vi "Steruerungs Type erkennen.vi"(8 "error in (no error)":errorcluster caption="Fehler (Eingang, kein Fehler)", 10 "Steuerungs Type":i32[](array[numeric]), 11 "Steuerung PNS Eingang":refnum<class "Steuerung PNS.lvclass">) -> (0 "error out":errorcluster caption="Fehler (Ausgang)", 3 "Steuerung PNS Ausgang":refnum<class "Steuerung PNS.lvclass">)   [LabVIEW 2020, in "Steuerung PNS.lvclass"]
doc: "Hier wird tatsächlich die OjektKlasse je nach SteuerungsType gewechselt und schreibt diese ins Objekt (falls diese noch nicht gesetzt wrude oder nicht mehr den selben Wert hat - Tausch des PNS mit AutoDetection).\nRIW"
uses:
  Steuerung PNS.lvclass
  Steuerung PNS.lvclass/Steuerung PNS.ctl
  SteuerungsType (Enum).ctl
  Schneider Steuerung PNS/Schneider Steuerung PNS.lvclass
  D:/LabView_2020/LP und Compact Standardprogramm_20-10-14/ObjektKlassen/Steuerung PNS/Steuerung PNS.lvclass
  mini8 Steuerung PNS/mini8 Steuerung PNS.lvclass
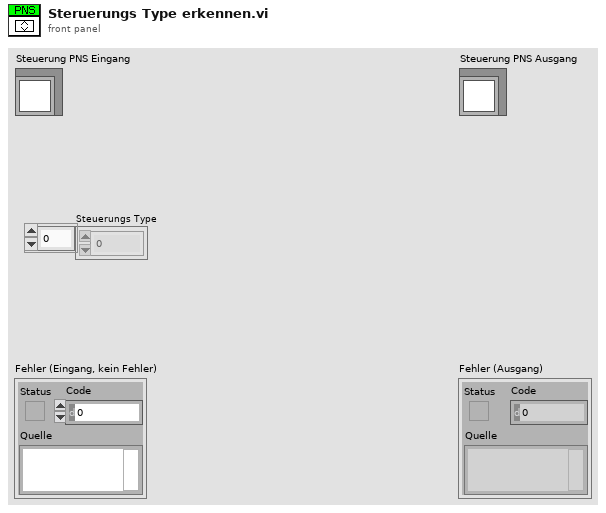
[diagram p1: front panel]
types:
  T1 = typedef "Steuerung PNS.lvclass/SteuerungsType (Enum).ctl" = enum16{"undefiniert", "Mini 8", "Schneider"}
  T2 = typedef "Steuerung PNS.lvclass/Anlegengrenzwerte PNS.ctl" = cluster{"Filter:":T3, "Ventilplatte:":T3, "Heizleitung 1:":T3, "Heizleitung 2:":T3, "Heizleitung 3:":T3, "Heizleitung 4:":T3, "Heizleitung 5:":T3, "Heizleitung 6:":T3}
  T3 = typedef "Steuerung PNS.lvclass/Anlagengrenzwerte Parameteranzeige.ctl" = cluster{"Sollwert":T4, "Warn-Min":T4, "Warn-Max":T4, "Abschalt-Min":T4, "Abschalt-Max":T4, "Regler":u16, "AnlagenParameter":string}
  T4 = typedef "Zahlen-Eingabefeld.ctl" = sgl
  T5 = typedef "Steuerung PNS.lvclass/Adresse.ctl" = cluster{i32[][], i32}
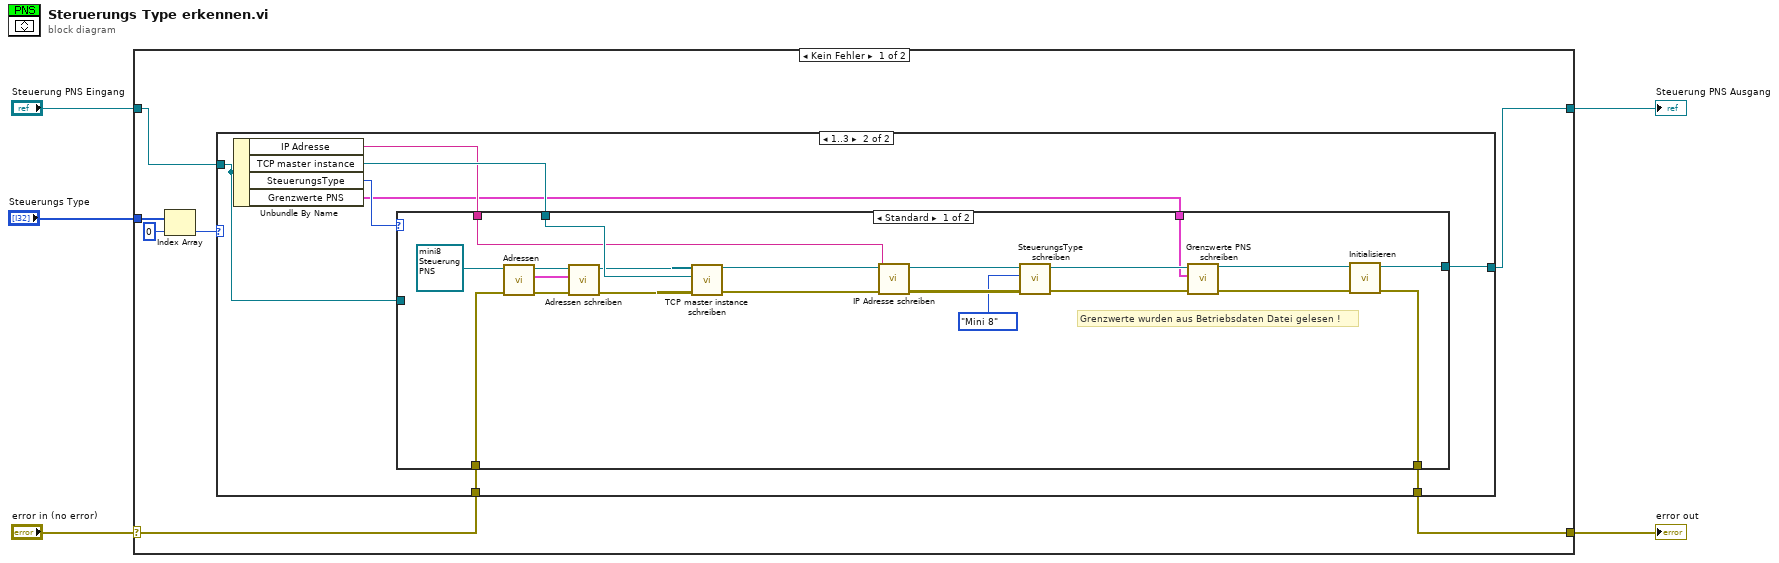
[diagram p0: block diagram]
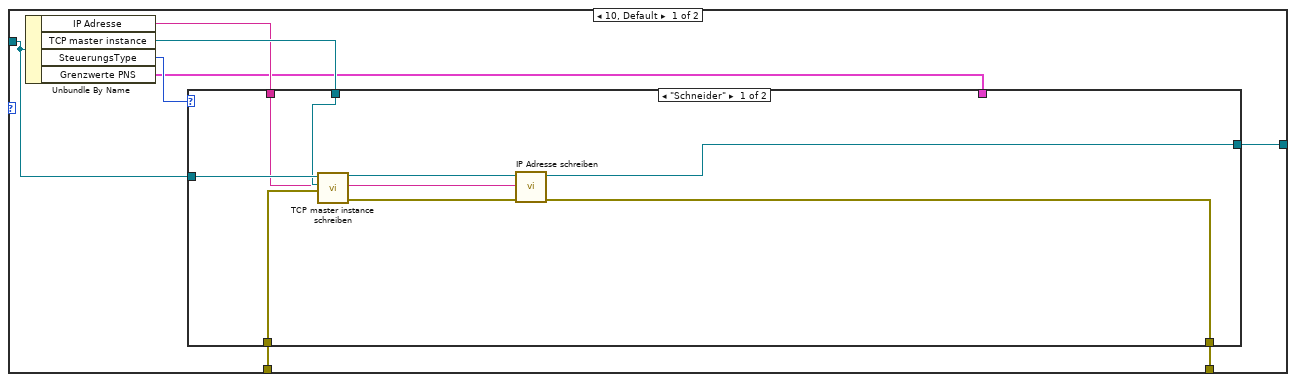
[diagram p2: hidden frame]
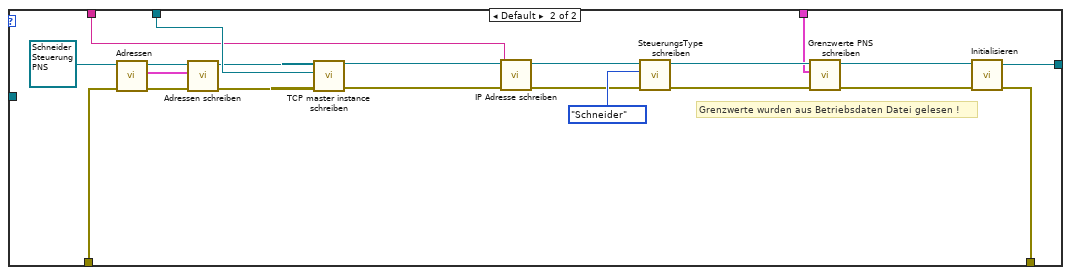
[diagram p3: hidden frame]
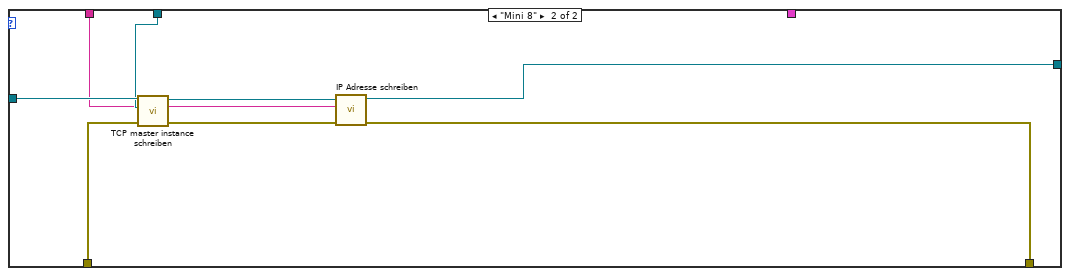
[diagram p4: hidden frame]
diagram:
  n1 = case shown="Kein Fehler" "error in (no error)" {
    selector: "error in (no error)" -> [w8 w86]
    tunnel: [w7 w86] -> w4
    tunnel: [w6 w85] -> w2
    tunnel: "Steuerung PNS Eingang" -> [w9 w85]
    tunnel: "Steuerungs Type" -> [w11 _]
    frame No Error {
      n2 = Index Array(array=w11, index=0 ("Index")) -> (element=w10:i32)
      n3 = case shown="1..3" w10 {
        tunnel: w9 -> [w14 w50]
        tunnel: w8 -> [w16 w52]
        tunnel: [w18 w56] -> w7
        tunnel: [w17 w53] -> w6
        frame 10, Default {
          n4 = Unbundle By Name(w14) -> ("IP Adresse"=w19:string, "TCP master instance"=w20:refnum<class "Modbus Master.lvclass">, "SteuerungsType"=w15:T1, "Grenzwerte PNS"=w13:T2)
          n5 = case shown="\"Schneider\"" w15 {
            tunnel: w20 -> [w22 w48]
            tunnel: w19 -> [w21 w29]
            tunnel: [w23 w39] -> w18
            tunnel: [w24 w38] -> w17
            tunnel: w16 -> [w26 w36]
            tunnel: w14 -> [w28 _]
            tunnel: w13 -> [_ w30]
            frame "Schneider" {
              n6 = call-dynamic "TCP master instance schreiben.vi"("error in (no error)"=w26, "Modbus Master"=w22, "Steuerung PNS (Eingang)"=w28) -> ("error out"=w25:errorcluster, "Steuerung PNS (Ausgang)"=w27:refnum<class "Steuerung PNS.lvclass">)  [unwired: 7 in]
              n7 = call-dynamic "IP Adresse schreiben.vi"("error in (no error)"=w25, "IP Adresse"=w21, "Steuerung PNS (Eingang)"=w27) -> ("error out"=w23:errorcluster, "Steuerung PNS (Ausgang)"=w24:refnum<class "Steuerung PNS.lvclass">)  [unwired: 7 in]
            }
            frame Default {
              # "Grenzwerte wurden aus Betriebsdaten Datei gelesen !"
              n8 = call-dynamic "Adressen.vi"("error in (no error)"=w36, "Schneider Steuerung PNS Eingang"=refnum<class "Schneider Steuerung PNS.lvclass"> refnum ("Schneider Steuerung PNS.lvclass")) -> ("error out"=w43:errorcluster, "Adressen out"=w44:T5, "Schneider Steuerung PNS Ausgang"=w45:refnum<class "Schneider Steuerung PNS.lvclass">)  [unwired: 7 in]
              n9 = call-dynamic "Adressen schreiben.vi"("error in (no error)"=w43, "Adressen"=w44, "Steuerung PNS (Eingang)"=w45) -> ("error out"=w32:errorcluster, "Steuerung PNS (Ausgang)"=w33:refnum<class "Schneider Steuerung PNS.lvclass">)  [unwired: 7 in]
              n10 = call-dynamic "TCP master instance schreiben.vi"("error in (no error)"=w32, "Modbus Master"=w48, "Steuerung PNS (Eingang)"=w33) -> ("error out"=w46:errorcluster, "Steuerung PNS (Ausgang)"=w47:refnum<class "Schneider Steuerung PNS.lvclass">)  [unwired: 7 in]
              n11 = call-dynamic "IP Adresse schreiben.vi"("error in (no error)"=w46, "IP Adresse"=w29, "Steuerung PNS (Eingang)"=w47) -> ("error out"=w34:errorcluster, "Steuerung PNS (Ausgang)"=w35:refnum<class "Schneider Steuerung PNS.lvclass">)  [unwired: 7 in]
              n12 = call-dynamic "SteuerungsType schreiben.vi"("error in (no error)"=w34, "SteuerungsType"=SteuerungsType_(Enum)."Schneider", "Steuerung PNS (Eingang)"=w35) -> ("error out"=w40:errorcluster, "Steuerung PNS (Ausgang)"=w41:refnum<class "Schneider Steuerung PNS.lvclass">)  [unwired: 7 in]
              n13 = call-dynamic "Grenzwerte PNS schreiben.vi"("Grenzwerte PNS"=w30, "Steuerung PNS (Eingang)"=w41) -> ("Steuerung PNS (Ausgang)"=w31:refnum<class "Schneider Steuerung PNS.lvclass">)  [unwired: 8 in, 1 out]
              n14 = call "Initialisieren.vi"("error in (no error)"=w40, "Steuerung PNS Eingang"=w31) -> ("error out"=w39:errorcluster, "Steuerung PNS Ausgang"=w38:refnum<class "Schneider Steuerung PNS.lvclass">)  [unwired: 8 in]
            }
          }
        }
        frame 1..3 {
          n15 = Unbundle By Name(w50) -> ("IP Adresse"=w54:string, "TCP master instance"=w55:refnum<class "Modbus Master.lvclass">, "SteuerungsType"=w51:T1, "Grenzwerte PNS"=w49:T2)
          n16 = case shown="Standard" w51 {
            tunnel: [w69 w80] -> w56
            tunnel: w55 -> [w68 w78]
            tunnel: w54 -> [w67 w77]
            tunnel: [w66 w79] -> w53
            tunnel: w52 -> [w61 w81]
            tunnel: w50 -> [_ w82]
            tunnel: w49 -> [w57 _]
            frame Default {
              # "Grenzwerte wurden aus Betriebsdaten Datei gelesen !"
              n17 = call-dynamic "Adressen.vi"("error in (no error)"=w61, "mini8 Steuerung PNS Eingang"=refnum<class "mini8 Steuerung PNS.lvclass"> refnum ("mini8 Steuerung PNS.lvclass")) -> ("error out"=w72:errorcluster, "Adressen out"=w73:T5, "mini8 Steuerung PNS Ausgang"=w74:refnum<class "mini8 Steuerung PNS.lvclass">)  [unwired: 7 in]
              n18 = call-dynamic "Adressen schreiben.vi"("error in (no error)"=w72, "Adressen"=w73, "Steuerung PNS (Eingang)"=w74) -> ("error out"=w59:errorcluster, "Steuerung PNS (Ausgang)"=w60:refnum<class "mini8 Steuerung PNS.lvclass">)  [unwired: 7 in]
              n19 = call-dynamic "TCP master instance schreiben.vi"("error in (no error)"=w59, "Modbus Master"=w68, "Steuerung PNS (Eingang)"=w60) -> ("error out"=w75:errorcluster, "Steuerung PNS (Ausgang)"=w76:refnum<class "mini8 Steuerung PNS.lvclass">)  [unwired: 7 in]
              n20 = call-dynamic "IP Adresse schreiben.vi"("error in (no error)"=w75, "IP Adresse"=w67, "Steuerung PNS (Eingang)"=w76) -> ("error out"=w65:errorcluster, "Steuerung PNS (Ausgang)"=w63:refnum<class "mini8 Steuerung PNS.lvclass">)  [unwired: 7 in]
              n21 = call-dynamic "SteuerungsType schreiben.vi"("error in (no error)"=w65, "SteuerungsType"=SteuerungsType_(Enum)."Mini 8", "Steuerung PNS (Eingang)"=w63) -> ("error out"=w70:errorcluster, "Steuerung PNS (Ausgang)"=w71:refnum<class "mini8 Steuerung PNS.lvclass">)  [unwired: 7 in]
              n22 = call-dynamic "Grenzwerte PNS schreiben.vi"("Grenzwerte PNS"=w57, "Steuerung PNS (Eingang)"=w71) -> ("Steuerung PNS (Ausgang)"=w58:refnum<class "mini8 Steuerung PNS.lvclass">)  [unwired: 8 in, 1 out]
              n23 = call "Initialisieren.vi"("error in (no error)"=w70, "Steuerung PNS Eingang"=w58) -> ("error out"=w69:errorcluster, "Steuerung PNS Ausgang"=w66:refnum<class "mini8 Steuerung PNS.lvclass">)  [unwired: 8 in]
            }
            frame "Mini 8" {
              n24 = call-dynamic "TCP master instance schreiben.vi"("error in (no error)"=w81, "Modbus Master"=w78, "Steuerung PNS (Eingang)"=w82) -> ("error out"=w83:errorcluster, "Steuerung PNS (Ausgang)"=w84:refnum<class "Steuerung PNS.lvclass">)  [unwired: 7 in]
              n25 = call-dynamic "IP Adresse schreiben.vi"("error in (no error)"=w83, "IP Adresse"=w77, "Steuerung PNS (Eingang)"=w84) -> ("error out"=w80:errorcluster, "Steuerung PNS (Ausgang)"=w79:refnum<class "Steuerung PNS.lvclass">)  [unwired: 7 in]
            }
          }
        }
      }
    }
    frame Error {
    }
  }
  "error out" <- w4
  "Steuerung PNS Ausgang" <- w2
